vi "Create APU Tree Layout.vi"(8 "error in (no error)":errorcluster, 10 "engine name":string, 11 "Section Ptr":T1 format="%.0x") -> (0 "error out":errorcluster, 2 "APU ref":T1 format="%.0x", 3 "Section Ptr dup":T1 format="%.0x")   [LabVIEW 2013, in "Engine Simulation Toolkit System Explorer.lvlib"]
uses:
  Engine Simulation Toolkit System Explorer.lvlib
  <vilib>/NI Veristand/Custom Device API/Custom Device Item Ref.ctl
  <vilib>/NI Veristand/Custom Device API/Custom Device Channel Type.ctl
  Shared/Constants and GUIDs.vi
  Shared/Properties.vi
  <vilib>/NI Veristand/Custom Device API/Set Item Property (String).vi
  <vilib>/NI Veristand/Custom Device API/Custom Device API.lvlib
  Shared/Engine Simulation Toolkit Shared.lvlib
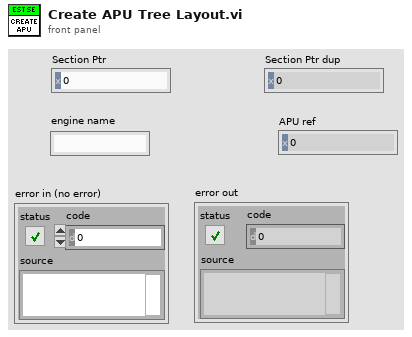
[diagram p1: front panel]
types:
  T1 = typedef "Custom Device API.lvlib/Custom Device Item Ref.ctl" = u64
  T2 = typedef "Custom Device API.lvlib/Custom Device Channel Type.ctl" = enum16{"Input", "Output"}
  T3 = typedef "Engine Simulation Toolkit Shared.lvlib/Channel.ctl" = cluster{"Name":string, "Units":string, "Default":dbl, "Description":string}
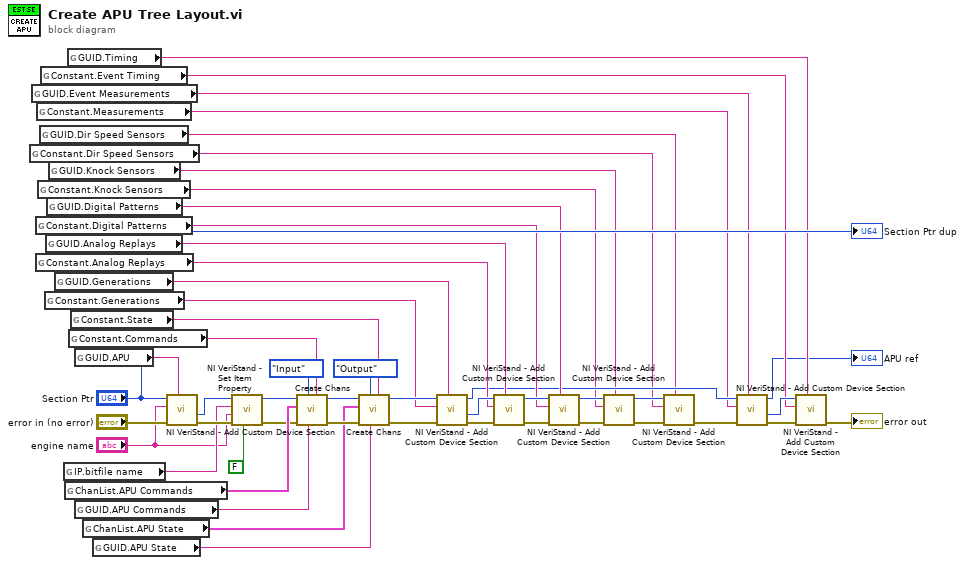
[diagram p0: block diagram]
diagram:
  n1 = global read "Constants and GUIDs.vi" "Constant.Dir Speed Sensors"() -> (w1:string)
  n2 = global read "Constants and GUIDs.vi" "GUID.Event Measurements"() -> (w20:string)
  n3 = global read "Constants and GUIDs.vi" "Constant.Digital Patterns"() -> (w26:string)
  n4 = global read "Constants and GUIDs.vi" "Constant.Analog Replays"() -> (w30:string)
  n5 = global read "Constants and GUIDs.vi" "Constant.Measurements"() -> (w23:string)
  n6 = global read "Constants and GUIDs.vi" "Constant.Knock Sensors"() -> (w5:string)
  n7 = global read "Constants and GUIDs.vi" "GUID.Dir Speed Sensors"() -> (w2:string)
  n8 = global read "Constants and GUIDs.vi" "Constant.Event Timing"() -> (w19:string)
  n9 = global read "Constants and GUIDs.vi" "Constant.Generations"() -> (w34:string)
  n10 = global read "Constants and GUIDs.vi" "GUID.Analog Replays"() -> (w29:string)
  n11 = global read "Constants and GUIDs.vi" "GUID.Digital Patterns"() -> (w25:string)
  n12 = global read "Constants and GUIDs.vi" "GUID.Knock Sensors"() -> (w6:string)
  n13 = global read "Constants and GUIDs.vi" "GUID.Generations"() -> (w33:string)
  n14 = global read "Properties.vi" "IP.bitfile name"() -> (w13:string)
  n15 = global read "Constants and GUIDs.vi" "ChanList.APU Commands"() -> (w44:T3[])
  n16 = global read "Constants and GUIDs.vi" "GUID.Timing"() -> (w18:string)
  n17 = global read "Constants and GUIDs.vi" "Constant.Commands"() -> (w45:string)
  n18 = global read "Constants and GUIDs.vi" "Constant.State"() -> (w39:string)
  n19 = global read "Constants and GUIDs.vi" "GUID.APU"() -> (w49:string)
  n20 = global read "Constants and GUIDs.vi" "GUID.APU Commands"() -> (w36:string)
  n21 = global read "Constants and GUIDs.vi" "ChanList.APU State"() -> (w41:T3[])
  n22 = global read "Constants and GUIDs.vi" "GUID.APU State"() -> (w35:string)
  n23 = call <vilib>:"NI VeriStand - Add Custom Device Section.vi"("GUID (Default Section)"=w49, "error in (no error)"="error in (no error)", "Section Name"="engine name", "Parent Ref in"="Section Ptr") -> ("error out"=w47:errorcluster, "Section Ptr"=w15:T1)  [unwired: 4 in, 2 out]
  n24 = call-poly <vilib>:"NI VeriStand - Set Item Property.vi"("Binary String (T)"=FALSE, "error in (no error)"=w47, "Value"="engine name", "Property Name"=w13, "Item Ref in"=w15) -> ("error out"=w16:errorcluster, "Item Ref out"=w14:T1)  [unwired: 4 in, 1 out]
  n25 = call "Create Chans.vi"("New Section Name (none)"=w45, "new section GUID (\"\":del prot)"=w36, "Type"=Custom_Device_Channel_Type."Input", "error in (no error)"=w16, "Channels"=w44, "Section Ptr"=w14) -> ("error out"=w43:errorcluster, "Section Ptr dup"=w42:T1)  [unwired: 2 in, 2 out]
  n26 = call "Create Chans.vi"("New Section Name (none)"=w39, "new section GUID (\"\":del prot)"=w35, "Type"=Custom_Device_Channel_Type."Output", "error in (no error)"=w43, "Channels"=w41, "Section Ptr"=w42) -> ("error out"=w38:errorcluster, "Section Ptr dup"=w37:T1)  [unwired: 2 in, 2 out]
  n27 = call <vilib>:"NI VeriStand - Add Custom Device Section.vi"("GUID (Default Section)"=w33, "error in (no error)"=w38, "Section Name"=w34, "Parent Ref in"=w37) -> ("error out"=w32:errorcluster, "Section Ptr"=w31:T1, "Parent Ref out"=w24:T1)  [unwired: 4 in, 1 out]
  n28 = call <vilib>:"NI VeriStand - Add Custom Device Section.vi"("GUID (Default Section)"=w29, "error in (no error)"=w32, "Section Name"=w30, "Parent Ref in"=w31) -> ("error out"=w28:errorcluster, "Parent Ref out"=w27:T1)  [unwired: 4 in, 2 out]
  n29 = call <vilib>:"NI VeriStand - Add Custom Device Section.vi"("GUID (Default Section)"=w25, "error in (no error)"=w28, "Section Name"=w26, "Parent Ref in"=w27) -> ("error out"=w9:errorcluster, "Parent Ref out"=w8:T1)  [unwired: 4 in, 2 out]
  n30 = call <vilib>:"NI VeriStand - Add Custom Device Section.vi"("GUID (Default Section)"=w6, "error in (no error)"=w9, "Section Name"=w5, "Parent Ref in"=w8) -> ("error out"=w7:errorcluster, "Parent Ref out"=w3:T1)  [unwired: 4 in, 2 out]
  n31 = call <vilib>:"NI VeriStand - Add Custom Device Section.vi"("GUID (Default Section)"=w2, "error in (no error)"=w7, "Section Name"=w1, "Parent Ref in"=w3) -> ("error out"=w4:errorcluster)  [unwired: 4 in, 3 out]
  n32 = call <vilib>:"NI VeriStand - Add Custom Device Section.vi"("GUID (Default Section)"=w20, "error in (no error)"=w4, "Section Name"=w23, "Parent Ref in"=w24) -> ("error out"=w22:errorcluster, "Section Ptr"=w21:T1, "Parent Ref out"=→"APU ref":T1)  [unwired: 4 in, 1 out]
  n33 = call <vilib>:"NI VeriStand - Add Custom Device Section.vi"("GUID (Default Section)"=w18, "error in (no error)"=w22, "Section Name"=w19, "Parent Ref in"=w21) -> ("error out"=→"error out":errorcluster)  [unwired: 4 in, 3 out]
  "Section Ptr dup" <- "Section Ptr"
